vi "DSF.Shared.Configuration.Transfer.Required Buffer Size.vi"(8 "error in (no error)":errorcluster, 11 "Transfer Configuration in":refnum<class "DSF.Shared.Configuration.Transfer.lvclass">) -> (0 "error out":errorcluster, 2 "required buffer size":u64 format="%d bytes", 3 "Transfer Configuration out":refnum<class "DSF.Shared.Configuration.Transfer.lvclass">)   [LabVIEW 2016, in "DSF.Shared.lvlib" / "DSF.Shared.Configuration.Transfer.lvclass"]
uses:
  DSF.Shared.Configuration.Transfer.lvclass
  DSF.Shared.Configuration.Transfer.lvclass/DSF.Shared.Configuration.Transfer.ctl
  VIs/DSF.Shared.Data Type.Sizeof.vi
  DSF.Shared.lvlib
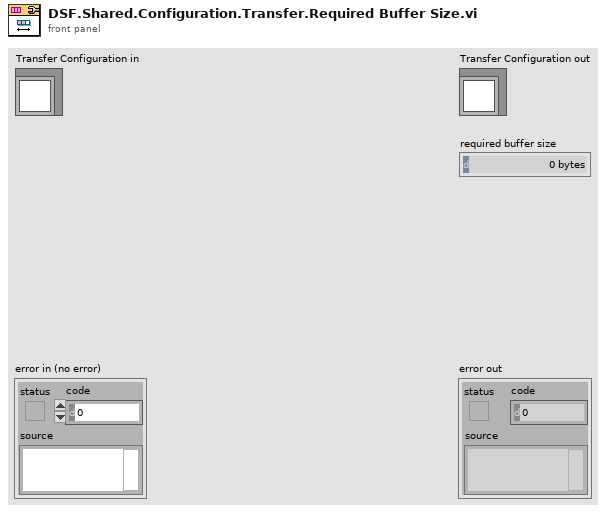
[diagram p1: front panel]
types:
  T1 = typedef "DSF.Shared.lvlib/DSF.Shared.Typedefs.Configuration.Transfer.Channel Block Descriptor.ctl" = cluster{"First Channel Descriptor":T2, "count":u64, "vs channel index":u64}
  T2 = typedef "DSF.Shared.lvlib/DSF.Shared.Typedefs.Configuration.Transfer.Channel Descriptor.ctl" = cluster{"Channel Parameters":T3, "VS Channel Ref":T5}
  T3 = typedef "DSF.Shared.lvlib/DSF.Shared.Typedefs.Configuration.Transfer.Channel Parameters.ctl" = cluster{"offset":u64, "data type":T4}
  T4 = typedef "DSF.Shared.lvlib/DSF.Shared.Typedefs.Data Type.ctl" = enum8{"Bool", "SGL", "DBL", "I8", "I16", "I32", "I64", "U8", "U16", "U32", "U64"}
  T5 = typedef "Custom Device API.lvlib/Custom Device Item Ref.ctl" = u64
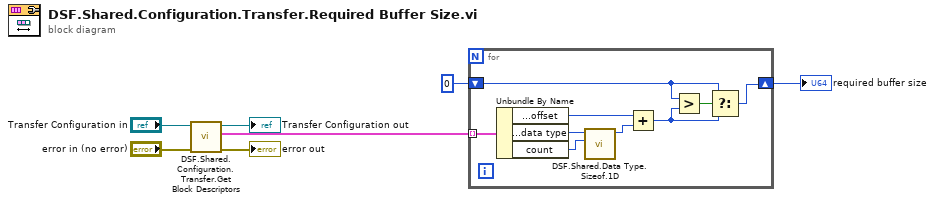
[diagram p0: block diagram]
diagram:
  n1 = call "DSF.Shared.Configuration.Transfer.Get Block Descriptors.vi"("Transfer Configuration in"="Transfer Configuration in") -> ("Channel Blocks"=w5:T1[], "Transfer Configuration out"=→"Transfer Configuration out":refnum<class "DSF.Shared.Configuration.Transfer.lvclass">)  [unwired: 9 in]
  n2 = for {
    tunnel: w5 -> [w15] mode=indexing
    shift-right: [w10] -> w2
    shift-left: u64 0 ("First Channel Descriptor.Channel Parameters.offset") -> [w7]
    n3 = Unbundle By Name(w15) -> ("First Channel Descriptor.Channel Parameters.offset"=w12:u64, "First Channel Descriptor.Channel Parameters.data type"=w14:T4, "count"=w13:u64)
    n4 = call "DSF.Shared.Data Type.Sizeof.1D.vi"("count"=w13, "data type"=w14) -> ("size in bytes"=w11:u64)  [unwired: 9 in]
    n5 = Add(x=w12, y=w11) -> (x+y=w8:u64)
    n6 = Greater?(x=w7, y=w8) -> (0:w9:bool)
    n7 = Select(t=w7, s=w9, f=w8) -> (s? t:f=w10:u64)
  }
  "required buffer size" <- w2
  "error out" <- "error in (no error)"
